vi "refModelRudder.vi"(10 "delta_d":dbl) -> (2 "delta_r":dbl)   [LabVIEW 2014]
uses:
  <vilib>/Simulation/Implementation/Shared/SIMSCR Execution Mode.ctl
  <vilib>/Simulation/Scripting/Companion Diagram/SimConfigNode/SimParams.ctl
  <vilib>/Simulation/Scripting/Companion Diagram/SimConfigNode/_simSolvers.ctl
  <vilib>/Simulation/Param Hierarchy/Typedefs/SIMPH Param Control Actions.ctl
  <vilib>/Simulation/Implementation/Shared/SIM limit type.ctl
  <vilib>/Simulation/Implementation/Shared/NILVSim_ParamChanged.vi
  <vilib>/Simulation/Implementation/Shared/NILVSIM_BeginStep.vi
  <vilib>/Simulation/ContinuousLinear/Implementation/NILVSim Integrator new.llb/SIM Integrator distributor (scalar).vi
  <vilib>/Simulation/SignalArithmetic/Implementation/NILVSim Gain.llb/SIM Gain (scalar).vi
  <vilib>/Simulation/Nonlinear/Implementation/NILVSim Saturation.llb/SIM Saturation (scalar).vi
  <vilib>/Simulation/ContinuousLinear/Implementation/NILVSim Integrator new.llb/SIM Integrator collector (scalar).vi
  <vilib>/Simulation/Implementation/Shared/NILVSim_Manager.vi
  <vilib>/Utility/error.llb/Clear Errors.vi
  <vilib>/Simulation/Implementation/Shared/NILVSim_FinalizeModel.vi
  <vilib>/Simulation/Implementation/Shared/SIM Unbundle Sim Info.vi
  <vilib>/Simulation/Implementation/Shared/SIMSH Read Queue.vi
  <vilib>/Simulation/Implementation/Shared/NILVSim_Initialize.vi
  <vilib>/Simulation/Utility/Implementation/NILVSim Get Time and IsAcceptedStep.vi
  <vilib>/Simulation/Implementation/Shared/NILVSim_GetModelError.vi
  <vilib>/Simulation/Implementation/Shared/SIM SimErrorHandler.vi
  <vilib>/Simulation/Implementation/Shared/SIM Bundle Sim Info.vi
  <vilib>/Simulation/Scripting/Companion Diagram/SimConfigNode/SimDog.xnode
  <vilib>/Simulation/Implementation/XNodeFramework/SimXNode/SimX.xnode
  <vilib>/Simulation/ContinuousLinear/Implementation/NILVSim Integrator new.llb/SIM Integrator (scalar).vi
  <vilib>/Simulation/Implementation/Shared/NI_SIM_Implementation.lvlib
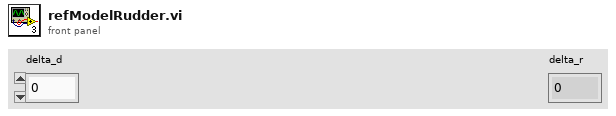
[diagram p1: front panel]
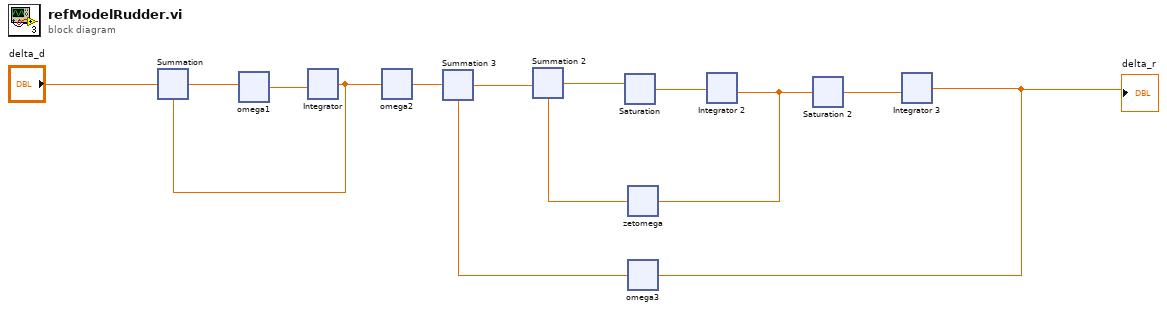
[diagram p0: block diagram]
diagram:
  n1 = xnode "Summation"("Operand1"="delta_d", "Operand2"=w3) -> ("Result"=w12:dbl)
  n2 = xnode "omega1"("input"=w12) -> ("output"=w11:dbl)  [unwired: 3 in]
  n3 = xnode "Integrator"("input"=w11) -> ("output"=w3:dbl)  [unwired: 9 in, 2 out]
  n4 = xnode "omega2"("input"=w3) -> ("output"=w2:dbl)  [unwired: 3 in]
  n5 = xnode "Summation 3"("Operand1"=w2, "Operand2"=w4) -> ("Result"=w1:dbl)
  n6 = xnode "Summation 2"("Operand1"=w1, "Operand2"=w6) -> ("Result"=w10:dbl)
  n7 = xnode "Saturation"("input"=w10) -> ("output"=w9:dbl)  [unwired: 4 in]
  n8 = xnode "Integrator 2"("input"=w9) -> ("output"=w7:dbl)  [unwired: 9 in, 2 out]
  n9 = xnode "zetomega"("input"=w7) -> ("output"=w6:dbl)  [unwired: 3 in]
  n10 = xnode "Saturation 2"("input"=w7) -> ("output"=w8:dbl)  [unwired: 4 in]
  n11 = xnode "Integrator 3"("input"=w8) -> ("output"=w5:dbl)  [unwired: 9 in, 2 out]
  "delta_r" <- w5
  n12 = xnode "omega3"("input"=w5) -> ("output"=w4:dbl)  [unwired: 3 in]
